vi "Set Column Widths (STUB).vi"(8 "error in (no error)":errorcluster, 11 "Tree Refnum":refnum<vi>) -> (0 "error out":errorcluster)   [LabVIEW 2015, in "TreeExtensions.lvlib"]
uses:
  TreeExtensions.lvlib
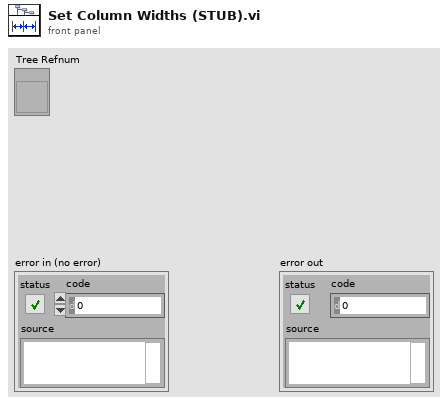
[diagram p1: front panel]
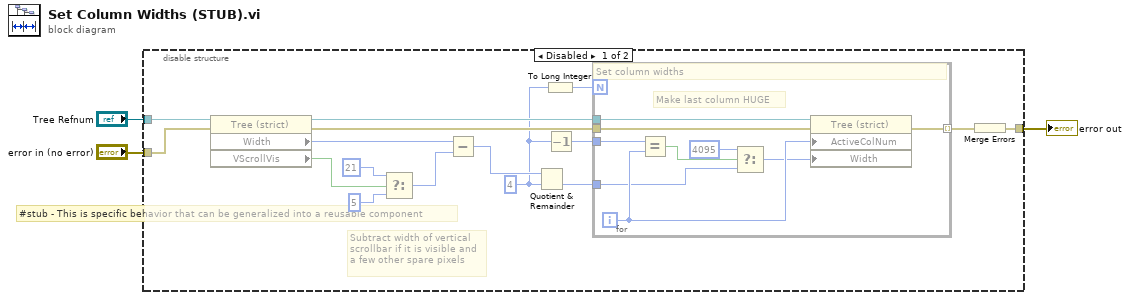
[diagram p0: block diagram]
diagram:
  # "#stub - This is specific behavior that can be generalized into a reusable component"
  n1 = disable-structure shown="Disabled" {
    disable-tunnel: "Tree Refnum" -> [w7 _]
    disable-tunnel: "error in (no error)" -> [w6 w29]
    disable-tunnel: [w4 w29] -> w1
    frame Disabled {
      w9 = u32 4 ("y")
      # "Subtract width of vertical\nscrollbar if it is visible and\na few other spare pixels"
      n2 = property class="Tree (strict)"(reference=w7, error in=w6) -> (reference out=w17:refnum<vi>, error out=w19:errorcluster, "Width"=w16:u32, "VScrollVis"=w15:bool)
      n3 = Select(t=u32 21, s=w15, f=u32 5) -> (s? t:f=w11:u32)
      n4 = Subtract(x=w16, y=w11) -> (x-y=w12:u32)
      n5 = Quotient & Remainder(x=w12, y=w9) -> (floor(x/y)=w10:u32)  [unwired: 1 out]
      n6 = To Long Integer(number=w9) -> (32bit integer=w18:i32)
      n7 = Decrement(x=w9) -> (x-1=w8:u32)
      n8 = for {
        N: w18 -> [_]
        tunnel: w17 -> [w28]
        tunnel: w10 -> [w24]
        tunnel: w8 -> [w26]
        tunnel: w19 -> [w21]
        tunnel: [w20] -> w5 mode=indexing
        i -> [w27]
        # "Make last column HUGE"
        # "Set column widths"
        n9 = Equal?(x=w26, y=w27) -> (x = y?=w25:bool)
        n10 = Select(t=u32 4095, s=w25, f=w24) -> (s? t:f=w23:u32)
        n11 = property class="Tree (strict)"(reference=w28, error in=w21, "ActiveColNum"=w27, "Width"=w23) -> (error out=w20:errorcluster)  [unwired: 1 out]
      }
      n12 = Merge Errors(w5) -> (w4:errorcluster)
    }
    frame Enabled {
    }
  }
  "error out" <- w1
